vi "rhozero.vi"(11 "Array in":dbl[](array[numeric])) -> (3 "Array out":dbl[](array[numeric]))   [LabVIEW 2020]
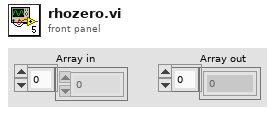
[diagram p1: front panel]
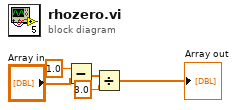
[diagram p0: block diagram]
diagram:
  n1 = Subtract(x=1.0, y="Array in") -> (x-y=w3:dbl[])
  n2 = Divide(x=w3, y=3.0) -> (x/y=→"Array out":dbl[])
